vi "Init Queue.vi"(8 "error in":errorcluster, 10 "queue_name":string, 11 "Instrument in":refnum<class "Instrument.lvclass">) -> (0 "error out":errorcluster, 3 "Instrument out":refnum<class "Instrument.lvclass">)   [LabVIEW 2018, in "Instrument.lvclass"]
doc: "Initialize the queue for state communication. The Instrument template uses a queued state machine to handle the current state. The initial state of the instrument is <B>Configure</B>. The queues will have unique names based upon the \"name\" provided by the child inheriting the class. If the name is not populated yet, then the queues may not be unique!"
uses:
  Instrument.lvclass
  state.ctl
  Instrument.lvclass/Instrument.ctl
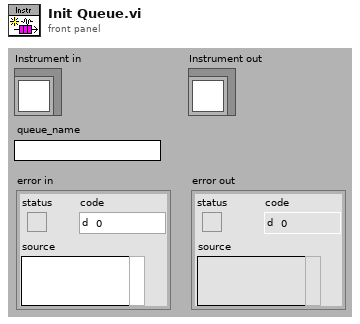
[diagram p1: front panel]
types:
  T1 = typedef "Instrument.lvclass/state.ctl" = enum8{"Configure", "Acquire", "Wait", "Quit", "Handle Error", "NOOP"}
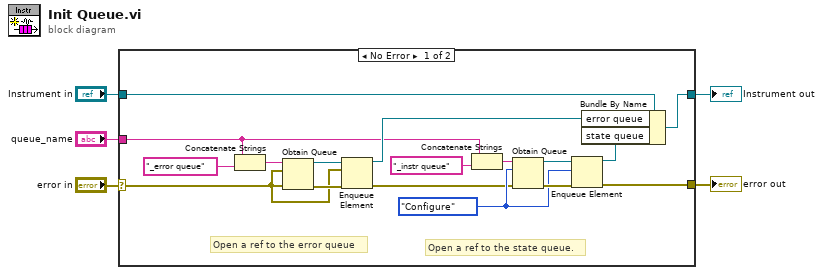
[diagram p0: block diagram]
diagram:
  n1 = case shown="No Error" "error in" {
    selector: "error in" -> [w15 w24]
    tunnel: [w12 w24] -> w4
    tunnel: [w22 w23] -> w2
    tunnel: "Instrument in" -> [w11 w23]
    tunnel: "queue_name" -> [w6 _]
    frame No Error {
      w19 = state."Configure" ("instr state")
      # "Open a ref to the state queue."
      # "Open a ref to the error queue"
      n2 = Concatenate Strings(w6, "_error queue" ("name (unnamed)")) -> (w9:string)
      n3 = Obtain Queue(name (unnamed)=w9, element data type=w15, error in (no error)=w15) -> (queue out=w17:refnum<queue>, error out=w16:errorcluster)  [unwired: 2 in, 1 out]
      n4 = Enqueue Element(queue=w17, element=w15, error in (no error)=w16) -> (queue out=w13:refnum<queue>, error out=w14:errorcluster)  [unwired: 1 in, 1 out]
      n5 = Concatenate Strings(w6, "_instr queue" ("name (unnamed)")) -> (w7:string)
      n6 = Obtain Queue(name (unnamed)=w7, element data type=w19, error in (no error)=w14) -> (queue out=w21:refnum<queue>, error out=w20:errorcluster)  [unwired: 2 in, 1 out]
      n7 = Enqueue Element(queue=w21, element=w19, error in (no error)=w20) -> (queue out=w18:refnum<queue>, error out=w12:errorcluster)  [unwired: 1 in, 1 out]
      n8 = Bundle By Name(cluster=w11, "error queue"=w13, "state queue"=w18) -> (w22:refnum<class "Instrument.lvclass">)
    }
    frame Error {
    }
  }
  "error out" <- w4
  "Instrument out" <- w2
